vi "Read AI Channel Setting Value.vi"(8 "error in (no error)":errorcluster, 10 "Data in":string[][][](array[string])) -> (0 "error out":errorcluster, 2 "Instrument Config":T1={"AI Setting"={"Physical Channel"=[], "Name to assign"=[], "minimum value"=0.0, "maximum value"=10.0, "custom scale name"="", "rate"=5000.0, "samples per channel"=1000, "input terminal configuration"=-1, "units"=10348, "sample mode"=10123}, "DI Channel Setting"={"DI Channel"=[]}, "AO Channel Setting"={"AO Channel name"=[], "output terminal configuration"=enum."RSE", "minimum value"=-10.0, "maximum value"=10.0, "units"=enum."Volts", "name to assign"=[]}, "DO Channel Setting"={"DO Channel"=[]}} {"AO Channel Setting"."maximum value" format="%0.2f"; "AO Channel Setting"."minimum value" format="%0.2f"; "AI Setting"."sample mode" items=["Finite Samples"=10178, "Continuous Samples"=10123, "Hardware Timed Single Point"=12522]; "AI Setting"."units" items=["Volts"=10348, "From Custom Scale"=10065]; "AI Setting"."input terminal configuration" items=["Default"=-1, "RSE"=10083, "NRSE"=10078, "Differential"=10106, "Pseudodifferential"=12529]; "AI Setting"."rate" format="%#_13g"; "AI Setting"."maximum value" format="%#_13g"; "AI Setting"."minimum value" format="%#_13g"})   [LabVIEW 2016, in "DAQ Hardware.lvlib"]
uses:
  DAQ Hardware.lvlib
  Instrument Config.ctl
  User Interface/AI Channel Setting.ctl
  DI Channel Setting.ctl
  AO Channel Setting.ctl
  DO Channel Setting.ctl
  User Interface/User Interface.lvlib
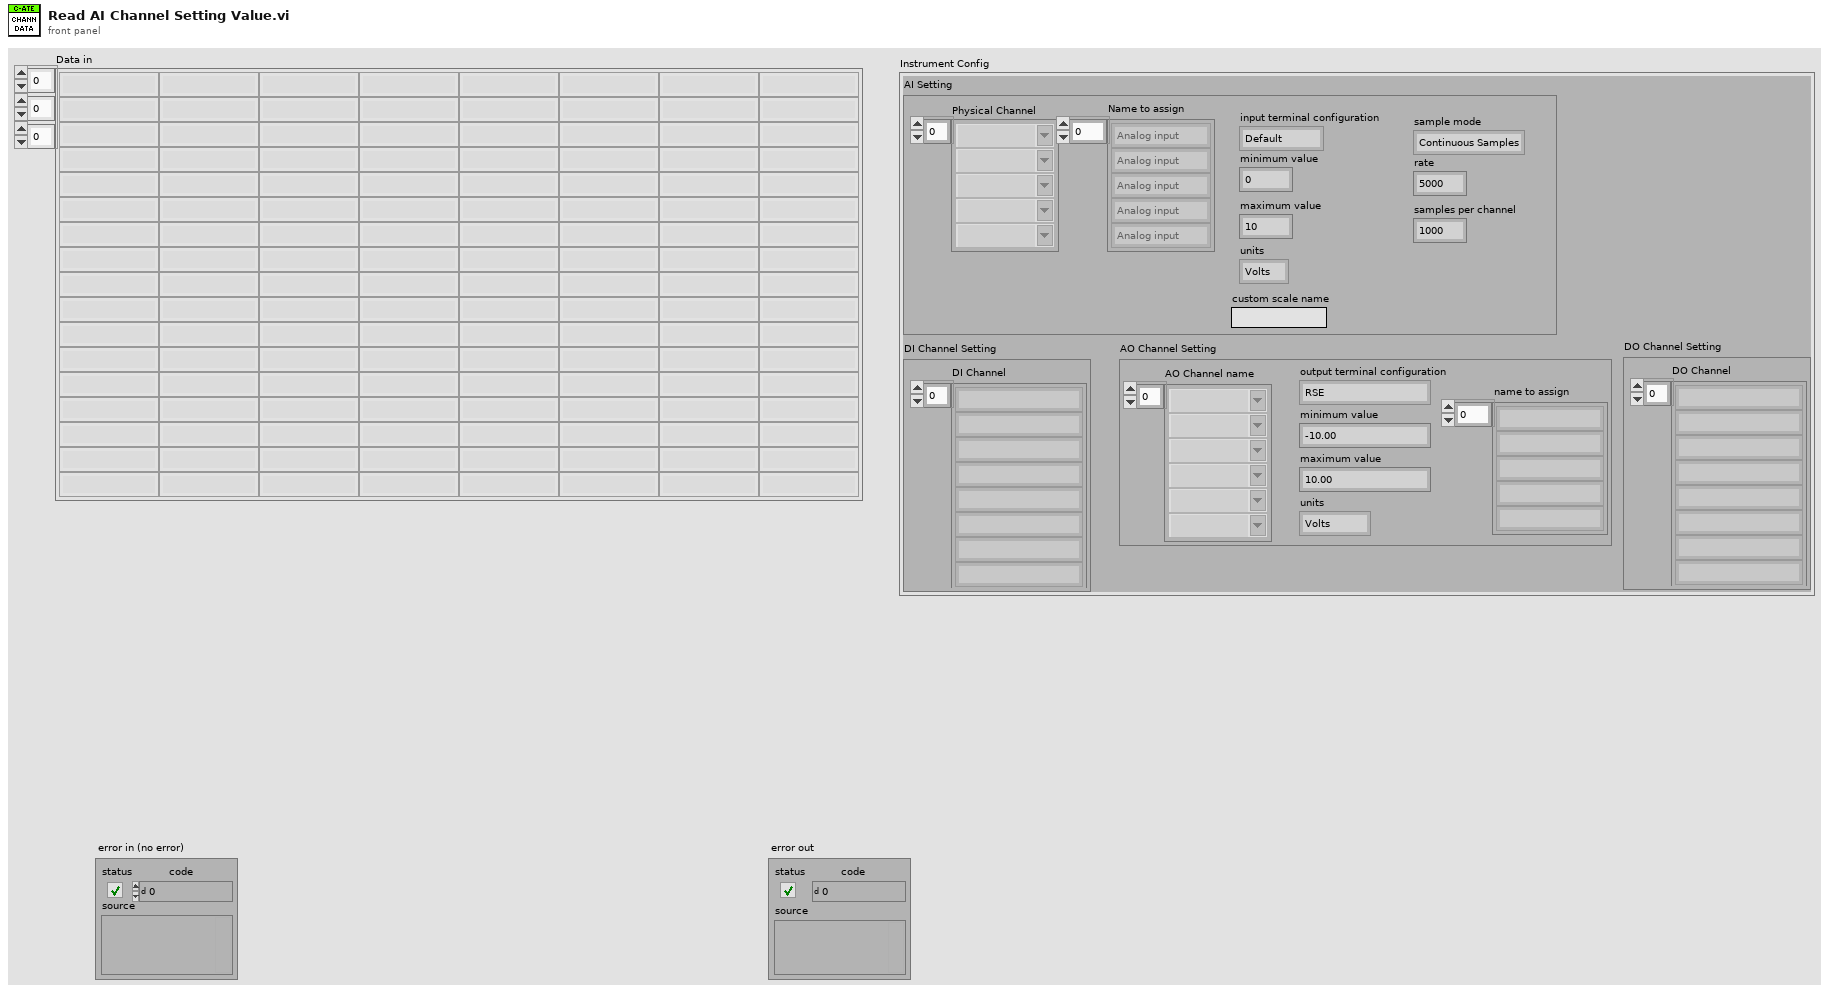
[diagram p1: front panel]
types:
  T1 = typedef "DAQ Hardware.lvlib/Instrument Config.ctl" = cluster{"AI Setting":T2, "DI Channel Setting":T3, "AO Channel Setting":T4, "DO Channel Setting":T5}
  T2 = typedef "DAQ Hardware.lvlib/AI Channel Setting.ctl" = cluster{"Physical Channel":string[], "Name to assign":string[], "minimum value":dbl, "maximum value":dbl, "custom scale name":string, "rate":dbl, "samples per channel":i32, "input terminal configuration":i32, "units":i32, "sample mode":i32}
  T3 = typedef "DAQ Hardware.lvlib/DI Channel Setting.ctl" = cluster{"DI Channel":string[]}
  T4 = typedef "DAQ Hardware.lvlib/AO Channel Setting.ctl" = cluster{"AO Channel name":string[], "output terminal configuration":enum16{"RSE", "NRSE", "Differential"}, "minimum value":dbl, "maximum value":dbl, "units":enum16{"Volts"}, "name to assign":string[]}
  T5 = typedef "DAQ Hardware.lvlib/DO Channel Setting.ctl" = cluster{"DO Channel":string[]}
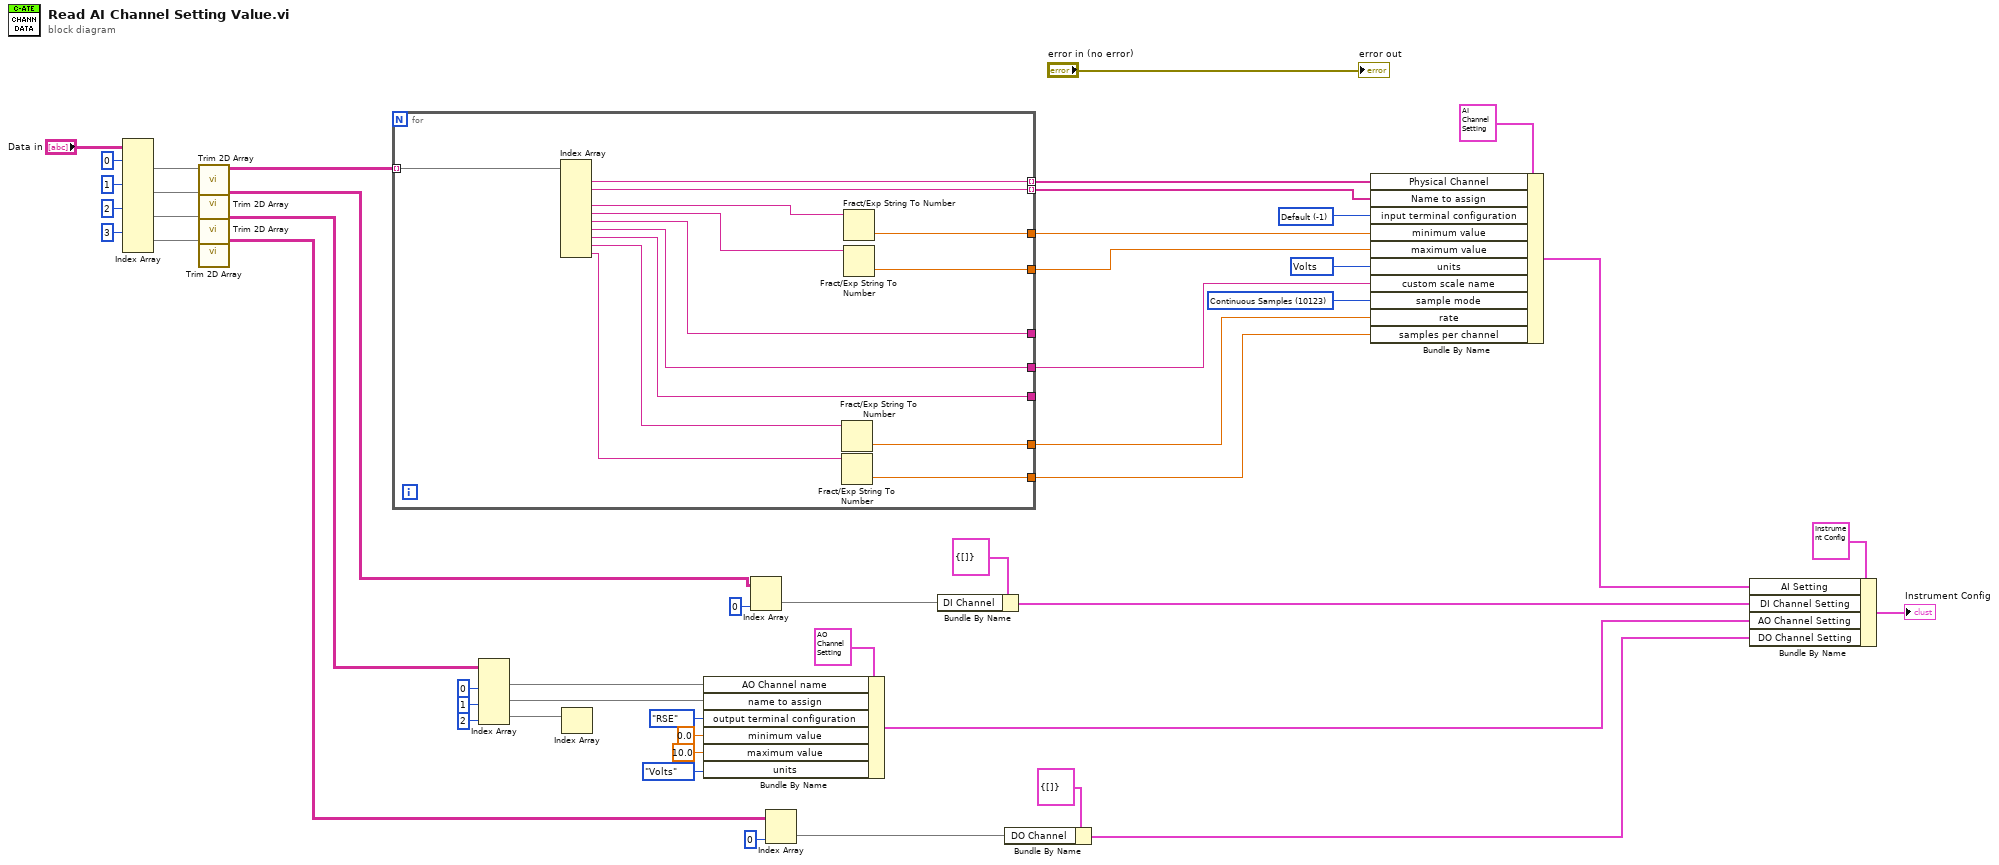
[diagram p0: block diagram]
diagram:
  w38 = 10123 items=["Finite Samples"=10178, "Continuous Samples"=10123, "Hardware Timed Single Point"=12522] ("sample mode")
  w41 = -1 items=["Default"=-1, "RSE"=10083, "NRSE"=10078, "Differential"=10106, "Pseudodifferential"=12529] ("input terminal configuration")
  w42 = 10348 items=["Volts"=10348, "From Custom Scale"=10065] ("units")
  n1 = Index Array(array="Data in", index (dim 0) #1=0 ("index (page)"), index (dim 0) #2=1 ("index (page)"), index (dim 0) #3=2 ("index (page)"), index (dim 0) #4=3 ("index (page)")) -> (element #1=w34:string[][], element #2=w31:string[][], element #3=w25:string[][], element #4=w6:string[][])  [unwired: 8 in]
  n2 = call "Trim 2D Array.vi"("Data in"=w34) -> ("Data out"=w33:string[][])  [unwired: 10 in]
  n3 = call "Trim 2D Array.vi"("Data in"=w31) -> ("Data out"=w26:string[][])  [unwired: 10 in]
  n4 = call "Trim 2D Array.vi"("Data in"=w25) -> ("Data out"=w24:string[][])  [unwired: 10 in]
  n5 = call "Trim 2D Array.vi"("Data in"=w6) -> ("Data out"=w3:string[][])  [unwired: 10 in]
  n6 = for {
    tunnel: w33 -> [w62] mode=indexing
    tunnel: [w61] -> w46 mode=indexing
    tunnel: [w60] -> w45 mode=indexing
    tunnel: [w59] -> w43
    tunnel: [w58] -> w44
    tunnel: [w57] -> _
    tunnel: [w56] -> w40
    tunnel: [w53] -> w39
    tunnel: [w50] -> _
    tunnel: [w49] -> w37
    n7 = Index Array(array=w62) -> (element #1=w61:string, element #2=w60:string, element #4=w52:string, element #5=w51:string, element #6=w57:string, element #7=w49:string, element #8=w50:string, element #9=w55:string, element #10=w54:string)  [unwired: 10 in, 1 out]
    n8 = Fract/Exp String To Number(string=w55) -> (number=w56:dbl)  [unwired: 3 in, 1 out]
    n9 = Fract/Exp String To Number(string=w54) -> (number=w53:dbl)  [unwired: 3 in, 1 out]
    n10 = Fract/Exp String To Number(string=w52) -> (number=w59:dbl)  [unwired: 3 in, 1 out]
    n11 = Fract/Exp String To Number(string=w51) -> (number=w58:dbl)  [unwired: 3 in, 1 out]
  }
  n12 = Index Array(array=w24, index (col) #1=0 ("disabled index (col)"), index (col) #2=1 ("index (col)"), index (col) #3=2 ("index (col)")) -> (element #1=w21:string[], element #2=w19:string[], element #3=w17:string[])  [unwired: 3 in]
  n13 = Index Array(array=w17) -> ()  [unwired: 1 in, 1 out]
  n14 = Bundle By Name(cluster=T4 {"AO Channel name"=[], "output terminal configuration"=enum."RSE", "minimum value"=-10.0, "maximum value"=10.0, "units"=enum."Volts", "name to assign"=[]} ("AO Channel Setting"), "AO Channel name"=w21, "name to assign"=w19, "output terminal configuration"=enum16{"RSE", "NRSE", "Differential"}."RSE", "minimum value"=0.0, "maximum value"=10.0, "units"=enum16{"Volts"}."Volts") -> (w9:T4)
  n15 = Index Array(array=w26, index (col)=0 ("disabled index (col)")) -> (element=w28:string[])  [unwired: 1 in]
  n16 = Index Array(array=w3, index (col)=0 ("disabled index (col)")) -> (element=w2:string[])  [unwired: 1 in]
  n17 = Bundle By Name(cluster=T3 {"DI Channel"=[]} ("DI Channel Setting"), "DI Channel"=w28) -> (w10:T3)
  n18 = Bundle By Name(cluster=T5 {"DO Channel"=[]} ("DO Channel Setting"), "DO Channel"=w2) -> (w1:T5)
  n19 = Bundle By Name(cluster=T2 {"Physical Channel"=["6363/ai0", "6363/ai1", "6363/ai2"], "Name to assign"=[], "minimum value"=0.0, "maximum value"=10.0, "custom scale name"="", "rate"=5000.0, "samples per channel"=1000, "input terminal configuration"=0, "units"=0, "sample mode"=0} ("AI Setting"), "Physical Channel"=w46, "Name to assign"=w45, "input terminal configuration"=w41, "minimum value"=w43, "maximum value"=w44, "units"=w42, "custom scale name"=w37, "sample mode"=w38, "rate"=w40, "samples per channel"=w39) -> (w11:T2)
  n20 = Bundle By Name(cluster=T1 {"AI Setting"={"Physical Channel"=[], "Name to assign"=[], "minimum value"=0.0, "maximum value"=10.0, "custom scale name"="", "rate"=5000.0, "samples per channel"=1000, "input terminal configuration"=-1, "units"=10348, "sample mode"=10123}, "DI Channel Setting"={"DI Channel"=[]}, "AO Channel Setting"={"AO Channel name"=[], "output terminal configuration"=enum."RSE", "minimum value"=-10.0, "maximum value"=10.0, "units"=enum."Volts", "name to assign"=[]}, "DO Channel Setting"={"DO Channel"=[]}}, "AI Setting"=w11, "DI Channel Setting"=w10, "AO Channel Setting"=w9, "DO Channel Setting"=w1) -> (→"Instrument Config":T1)
  "error out" <- "error in (no error)"
